vi "I2C Thermal Camera AMG8833 8x8.vi"() -> ()   [LabVIEW 2020, in "CTI-Scratchpad.lvlib"]
uses:
  CTI-Scratchpad.lvlib
  CTI/Identity.ctl
  CTI/Error Reporting.ctl
  CTI/GPIO Number.ctl
  CTI/I2C Number.ctl
  <vilib>/gmath/interp.llb/Interpolate 2D (2d X,Y).vi
  CTI/Session/Session.lvclass
  CTI-Peripheral/Thermal Camera/I2C Thermal Camera/AMG8833 8x8/AMG8833 8x8 Camera.lvclass
  CTI/VisaComms/VisaComms.lvclass
  CTI/CTI.lvlib
  <vilib>/gmath/NI_Gmath.lvlib
panel:
  in  "Colormap Name":T1(ring)=enum."inferno"
  out "Intensity Graph 2":dbl[][](graph)
  in  "method":i32(ring)=3 items=["nearest", "bilinear", "bicubic", "bicubic spline"]
  out "Intensity Graph":dbl[][](graph)
  in  "Stop":bool
  out "loop":i32
  out "Identity":T2
  in  "Grove Connector":enum16{"I2C0", "I2C1"}(ring)
  out "error out":errorcluster
  in  "Port":refnum<visa-resource-name>="COM9"
  # "https://wiki.seeedstudio.com/Grove-Infrared_Temperature_Sensor_Array-AMG8833/"
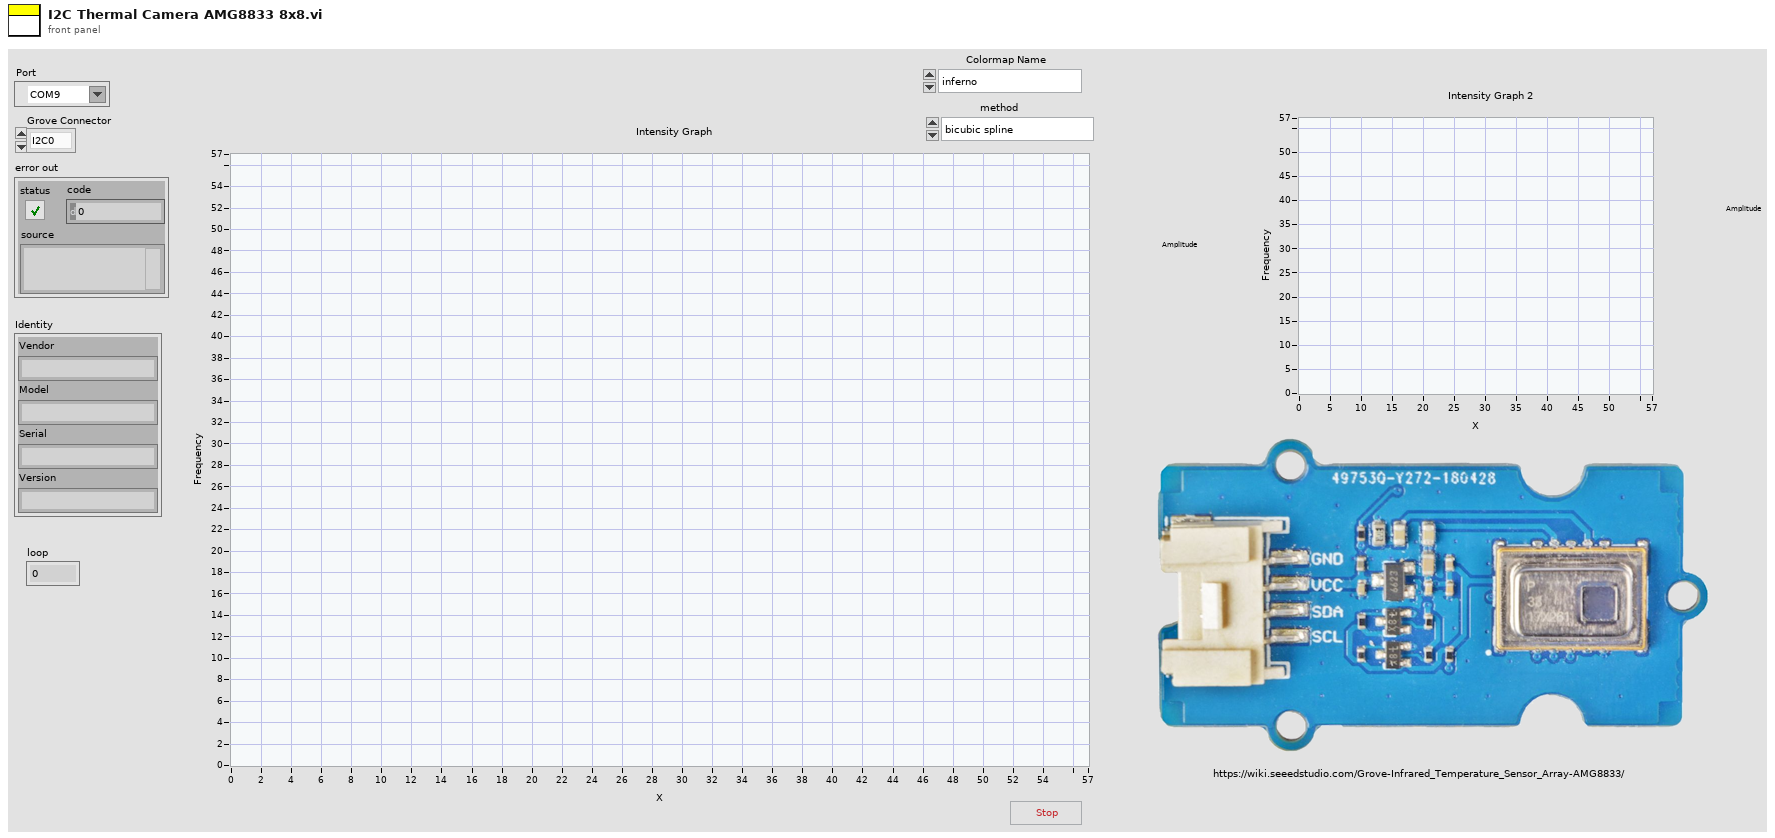
[diagram p1: front panel]
types:
  T1 = enum16{"magma", "inferno", "plasma", "viridis", "cividis", "twilight", "twilight_shifted", "turbo", "berlin", "managua", "vanimo"}
  T2 = typedef "CTI.lvlib/Identity.ctl" = cluster{"Vendor":string, "Model":string, "Serial":string, "Version":string}
  T3 = typedef "CTI.lvlib/Error Reporting.ctl" = enum16{"Minimal", "Moderate", "Full"}
  T4 = typedef "CTI.lvlib/I2C Number.ctl" = i8
  T5 = typedef "CTI.lvlib/GPIO Number.ctl" = i8
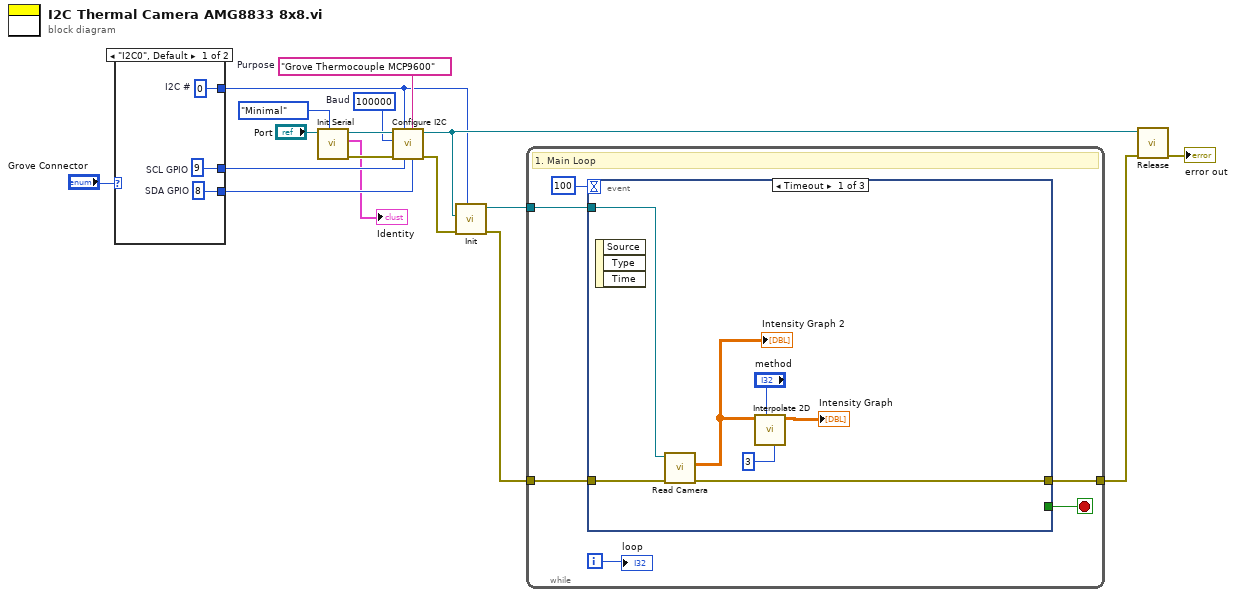
[diagram p0: block diagram]
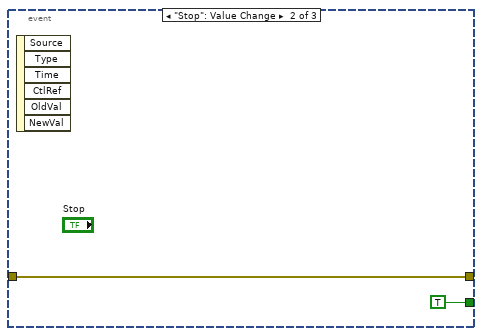
[diagram p2: hidden frame]
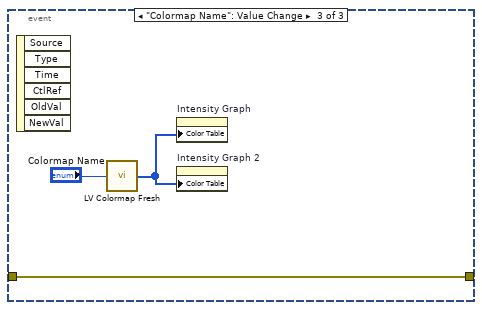
[diagram p3: hidden frame]
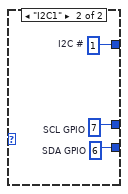
[diagram p4: hidden frame]
diagram:
  w12 = "Grove Thermocouple MCP9600"  # Purpose
  w13 = u32 100000  # Baud
  n1 = case shown="\"I2C0\", Default" "Grove Connector" {
    tunnel: [w20 w23] -> w8
    tunnel: [w19 w22] -> w7
    tunnel: [w18 w21] -> w6
    frame "I2C0", Default {
      w18 = T4 0  # I2C #
      w19 = T5 8  # SDA GPIO
      w20 = T5 9  # SCL GPIO
    }
    frame "I2C1" {
      w21 = T4 1  # I2C #
      w22 = T5 6  # SDA GPIO
      w23 = T5 7  # SCL GPIO
    }
  }
  n2 = call "Init Serial.vi"("Error Checking (Full)"=Error_Reporting."Minimal", "VISA resource name in"="Port") -> ("error out"=w14:errorcluster, "Identity"=→"Identity":T2, "Session"=w15:refnum<class "Session.lvclass">)  [unwired: 7 in]
  n3 = call "Configure I2C.vi"("SDA GPIO"=w7, "Purpose (\"I2C\")"=w12, "SCL GPIO"=w8, "I2C #"=w6, "error in (no error)"=w14, "Baud"=w13, "Session in"=w15) -> ("error out"=w11:errorcluster, "Session out"=w10:refnum<class "Session.lvclass">)  [unwired: 3 in]
  n4 = call "Init.vi"("I2C #"=w6, "error in (no error)"=w11, "Session In"=w10) -> ("error out"=w1:errorcluster, "AMG8833 8x8 Camera Out"=w4:refnum<class "AMG8833 8x8 Camera.lvclass">)  [unwired: 7 in]
  n5 = while {
    tunnel: w1 -> [w28]
    tunnel: w4 -> [w29]
    tunnel: [w26] -> w3
    i -> [w27]
    stop <- w24 stop-if-true
    # "1. Main Loop"
    n6 = event shown="[0] Timeout" {
      selector: _ -> [_ _ _]
      dyn-events: _ -> [_ _ _]
      timeout: 100 -> [_ _ _]
      tunnel: w29 -> [w35 _ _]
      tunnel: w28 -> [w36 w37 w41]
      tunnel: [w34 w37 w41] -> w26
      tunnel: [_ TRUE _] -> w24
      event Timeout {
        n7 = event-data() -> ()  [unwired: 1 in, 3 out]
        n8 = call-dynamic "Read Camera.vi"("error in (no error)"=w36, "AMG8833 8x8 Camera in"=w35) -> ("error out"=w34:errorcluster, "Camera Output"=w30:dbl[][])  [unwired: 7 in, 1 out]
        "Intensity Graph 2" <- w30
        n9 = call-poly <vilib>:"Interpolate 2D.vi"("ntimes"=3, "method"="method", "Z"=w30) -> ("zi"=→"Intensity Graph":dbl[][])  [unwired: 5 in, 3 out]
      }
      event "Stop": Value Change {
        n10 = event-data() -> ()  [unwired: 1 in, 6 out]
      }
      event "Colormap Name": Value Change {
        n11 = event-data() -> ()  [unwired: 1 in, 6 out]
        n12 = call "LV Colormap Fresh.vi"("Colormap Name"="Colormap Name") -> ("Colormap"=w39:u32[])  [unwired: 14 in]
        n13 = property on="Intensity Graph" class="IntGraph (strict)"("Color Table"=w39) -> ()  [unwired: 2 in, 2 out]
        n14 = property on="Intensity Graph 2" class="IntGraph (strict)"("Color Table"=w39) -> ()  [unwired: 2 in, 2 out]
      }
    }
    "loop" <- w27
  }
  n15 = call-dynamic "Release.vi"("error in (no error)"=w3, "Session in"=w10) -> ("error out"=→"error out":errorcluster)  [unwired: 9 in]
